vi "Trial Graphs.vi"() -> ()   [LabVIEW 2020, in "AoC 2022.lvlib"]
uses:
  <userlib>/_OpenG.lib/array/array.llb/Sort 1D Array (DBL)__ogtk.vi
  <userlib>/_OpenG.lib/array/array.llb/Index 1D Array Elements (DBL)__ogtk.vi
  AoC 2022.lvlib
  <vilib>/Analysis/NI_AAL_Geometry.lvlib
  <vilib>/4SmartMachines/Polygon Clipping/polyClipping.lvlib
panel:
  out "Polygon Set 1":T1(array[cluster])
  out "error out":errorcluster
  out "x+y 3":dbl format="%#_18f"
  out "Centroid Y":dbl format="%#_10f"
  out "Centroid X":dbl format="%#_10f"
  out "appended array":cluster{cluster{"X":dbl, "Y":dbl}[]}[](array[cluster]) {"?"."X" format="%#_17f"; "?"."Y" format="%#_17f"}
  out "x+y 2":dbl format="%#_18f"
  out "x+y":dbl format="%#_18f"
  out "element":cluster{"X":dbl, "Y":dbl} {"X" format="%#_6f"; "Y" format="%#_6f"}
  out "Array 4":T2(array[cluster])
  out "size(s) 3":i32
  out "size(s) 2":i32
  out "size(s)":i32
  in  "milliseconds to wait":u32
  out "Array 3":T2(array[cluster])
  out "Array 2":T3(array[cluster]) {"?"."Intersection X" format="%#_6f"; "?"."Intersection Y" format="%#_6f"}
  out "number of columns":i32
  out "number of rows":i32
  out "24-bit pixmap":u32[][](array[colorbox])
  out "XY Graph":cluster{"X":dbl[], "Y":dbl[]}[](graph)
  in  "Sensors":T4(c390)={{"X"=46556, "Y"=1283362}={"Beacon"={"X"=-91140, "Y"=1441882}, "Distance to Beacon"=296216.0, "Coverage Area"={"X"=[-249660.0, 46556.0, 342772.0, 46556.0, -249660.0], "Y"=[1283362.0, 987146.0, 1283362.0, 1579578.0, 1283362.0]}}, {"X"=117432, "Y"=1503889}={"Beacon"={"X"=-91140, "Y"=1441882}, "Distance to Beacon"=270579.0, "Coverage Area"={"X"=[-153147.0, 117432.0, 388011.0, 117432.0, -153147.0], "Y"=[1503889.0, 1233310.0, 1503889.0, 1774468.0, 1503889.0]}}, {"X"=117970, "Y"=37503}={"Beacon"={"X"=436611, "Y"=263737}, "Distance to Beacon"=544875.0, "Coverage Area"={"X"=[-426905.0, 117970.0, 662845.0, 117970.0, -426905.0], "Y"=[37503.0, -507372.0, 37503.0, 582378.0, 37503.0]}}, {"X"=193367, "Y"=2712458}={"Beacon"={"X"=-91140, "Y"=1441882}, "Distance to Beacon"=1555083.0, "Coverage Area"={"X"=[-1361716.0, 193367.0, 1748450.0, 193367.0, -1361716.0], "Y"=[2712458.0, 1157375.0, 2712458.0, 4267541.0, 2712458.0]}}, {"X"=220580, "Y"=684270}={"Beacon"={"X"=436611, "Y"=263737}, "Distance to Beacon"=636564.0, "Coverage Area"={"X"=[-415984.0, 220580.0, 857144.0, 220580.0, -415984.0], "Y"=[684270.0, 47706.0, 684270.0, 1320834.0, 684270.0]}}, {"X"=273443, "Y"=171076}={"Beacon"={"X"=436611, "Y"=263737}, "Distance to Beacon"=255829.0, "Coverage Area"={"X"=[17614.0, 273443.0, 529272.0, 273443.0, 17614.0], "Y"=[171076.0, -84753.0, 171076.0, 426905.0, 171076.0]}}, {"X"=480296, "Y"=3999646}={"Beacon"={"X"=1694700, "Y"=4178942}, "Distance to Beacon"=1393700.0, "Coverage Area"={"X"=[-913404.0, 480296.0, 1873996.0, 480296.0, -913404.0], "Y"=[3999646.0, 2605946.0, 3999646.0, 5393346.0, 3999646.0]}}, {"X"=608229, "Y"=955721}={"Beacon"={"X"=436611, "Y"=263737}, "Distance to Beacon"=863602.0, "Coverage Area"={"X"=[-255373.0, 608229.0, 1471831.0, 608229.0, -255373.0], "Y"=[955721.0, 92119.0, 955721.0, 1819323.0, 955721.0]}}, {"X"=766640, "Y"=26597}={"Beacon"={"X"=436611, "Y"=263737}, "Distance to Beacon"=567169.0, "Coverage Area"={"X"=[199471.0, 766640.0, 1333809.0, 766640.0, 199471.0], "Y"=[26597.0, -540572.0, 26597.0, 593766.0, 26597.0]}}, {"X"=856867, "Y"=3271314}={"Beacon"={"X"=1829362, "Y"=3182862}, "Distance to Beacon"=1060947.0, "Coverage Area"={"X"=[-204080.0, 856867.0, 1917814.0, 856867.0, -204080.0], "Y"=[3271314.0, 2210367.0, 3271314.0, 4332261.0, 3271314.0]}}, {"X"=915040, "Y"=1835970}={"Beacon"={"X"=-91140, "Y"=1441882}, "Distance to Beacon"=1400268.0, "Coverage Area"={"X"=[-485228.0, 915040.0, 2315308.0, 915040.0, -485228.0], "Y"=[1835970.0, 435702.0, 1835970.0, 3236238.0, 1835970.0]}}, {"X"=1136011, "Y"=261705}={"Beacon"={"X"=436611, "Y"=263737}, "Distance to Beacon"=701432.0, "Coverage Area"={"X"=[434579.0, 1136011.0, 1837443.0, 1136011.0, 434579.0], "Y"=[261705.0, -439727.0, 261705.0, 963137.0, 261705.0]}}, {"X"=1189379, "Y"=3999750}={"Beacon"={"X"=1694700, "Y"=4178942}, "Distance to Beacon"=684513.0, "Coverage Area"={"X"=[504866.0, 1189379.0, 1873892.0, 1189379.0, 504866.0], "Y"=[3999750.0, 3315237.0, 3999750.0, 4684263.0, 3999750.0]}}, {"X"=1531981, "Y"=3801761}={"Beacon"={"X"=1694700, "Y"=4178942}, "Distance to Beacon"=539900.0, "Coverage Area"={"X"=[992081.0, 1531981.0, 2071881.0, 1531981.0, 992081.0], "Y"=[3801761.0, 3261861.0, 3801761.0, 4341661.0, 3801761.0]}}, {"X"=1662543, "Y"=3128823}={"Beacon"={"X"=1829362, "Y"=3182862}, "Distance to Beacon"=220858.0, "Coverage Area"={"X"=[1441685.0, 1662543.0, 1883401.0, 1662543.0, 1441685.0], "Y"=[3128823.0, 2907965.0, 3128823.0, 3349681.0, 3128823.0]}}, {"X"=1728351, "Y"=2895399}={"Beacon"={"X"=1829362, "Y"=3182862}, "Distance to Beacon"=388474.0, "Coverage Area"={"X"=[1339877.0, 1728351.0, 2116825.0, 1728351.0, 1339877.0], "Y"=[2895399.0, 2506925.0, 2895399.0, 3283873.0, 2895399.0]}}, {"X"=1810202, "Y"=3423309}={"Beacon"={"X"=1829362, "Y"=3182862}, "Distance to Beacon"=259607.0, "Coverage Area"={"X"=[1550595.0, 1810202.0, 2069809.0, 1810202.0, 1550595.0], "Y"=[3423309.0, 3163702.0, 3423309.0, 3682916.0, 3423309.0]}}, {"X"=1844282, "Y"=2994285}={"Beacon"={"X"=1829362, "Y"=3182862}, "Distance to Beacon"=203497.0, "Coverage Area"={"X"=[1640785.0, 1844282.0, 2047779.0, 1844282.0, 1640785.0], "Y"=[2994285.0, 2790788.0, 2994285.0, 3197782.0, 2994285.0]}}, {"X"=1878117, "Y"=2578817}={"Beacon"={"X"=2197530, "Y"=2271330}, "Distance to Beacon"=626900.0, "Coverage Area"={"X"=[1251217.0, 1878117.0, 2505017.0, 1878117.0, 1251217.0], "Y"=[2578817.0, 1951917.0, 2578817.0, 3205717.0, 2578817.0]}}, {"X"=1894207, "Y"=1168355}={"Beacon"={"X"=2197530, "Y"=2271330}, "Distance to Beacon"=1406298.0, "Coverage Area"={"X"=[487909.0, 1894207.0, 3300505.0, 1894207.0, 487909.0], "Y"=[1168355.0, -237943.0, 1168355.0, 2574653.0, 1168355.0]}}, {"X"=2343111, "Y"=66183}={"Beacon"={"X"=2081841, "Y"=-807749}, "Distance to Beacon"=1135202.0, "Coverage Area"={"X"=[1207909.0, 2343111.0, 3478313.0, 2343111.0, 1207909.0], "Y"=[66183.0, -1069019.0, 66183.0, 1201385.0, 66183.0]}}, {"X"=2439089, "Y"=3168242}={"Beacon"={"X"=1829362, "Y"=3182862}, "Distance to Beacon"=624347.0, "Coverage Area"={"X"=[1814742.0, 2439089.0, 3063436.0, 2439089.0, 1814742.0], "Y"=[3168242.0, 2543895.0, 3168242.0, 3792589.0, 3168242.0]}}, {"X"=2482373, "Y"=2648092}={"Beacon"={"X"=2197530, "Y"=2271330}, "Distance to Beacon"=661605.0, "Coverage Area"={"X"=[1820768.0, 2482373.0, 3143978.0, 2482373.0, 1820768.0], "Y"=[2648092.0, 1986487.0, 2648092.0, 3309697.0, 2648092.0]}}, {"X"=2569893, "Y"=3911832}={"Beacon"={"X"=1694700, "Y"=4178942}, "Distance to Beacon"=1142303.0, "Coverage Area"={"X"=[1427590.0, 2569893.0, 3712196.0, 2569893.0, 1427590.0], "Y"=[3911832.0, 2769529.0, 3911832.0, 5054135.0, 3911832.0]}}, {"X"=2605308, "Y"=2023938}={"Beacon"={"X"=2197530, "Y"=2271330}, "Distance to Beacon"=655170.0, "Coverage Area"={"X"=[1950138.0, 2605308.0, 3260478.0, 2605308.0, 1950138.0], "Y"=[2023938.0, 1368768.0, 2023938.0, 2679108.0, 2023938.0]}}, {"X"=3047883, "Y"=3301452}={"Beacon"={"X"=3537901, "Y"=3368697}, "Distance to Beacon"=557263.0, "Coverage Area"={"X"=[2490620.0, 3047883.0, 3605146.0, 3047883.0, 2490620.0], "Y"=[3301452.0, 2744189.0, 3301452.0, 3858715.0, 3301452.0]}}, {"X"=3056788, "Y"=2626224}={"Beacon"={"X"=3355914, "Y"=2862466}, "Distance to Beacon"=535368.0, "Coverage Area"={"X"=[2521420.0, 3056788.0, 3592156.0, 3056788.0, 2521420.0], "Y"=[2626224.0, 2090856.0, 2626224.0, 3161592.0, 2626224.0]}}, {"X"=3199067, "Y"=2194575}={"Beacon"={"X"=3748004, "Y"=2000000}, "Distance to Beacon"=743512.0, "Coverage Area"={"X"=[2455555.0, 3199067.0, 3942579.0, 3199067.0, 2455555.0], "Y"=[2194575.0, 1451063.0, 2194575.0, 2938087.0, 2194575.0]}}, {"X"=3329538, "Y"=3016377}={"Beacon"={"X"=3355914, "Y"=2862466}, "Distance to Beacon"=180287.0, "Coverage Area"={"X"=[3149251.0, 3329538.0, 3509825.0, 3329538.0, 3149251.0], "Y"=[3016377.0, 2836090.0, 3016377.0, 3196664.0, 3016377.0]}}, {"X"=3399994, "Y"=700264}={"Beacon"={"X"=3748004, "Y"=2000000}, "Distance to Beacon"=1647746.0, "Coverage Area"={"X"=[1752248.0, 3399994.0, 5047740.0, 3399994.0, 1752248.0], "Y"=[700264.0, -947482.0, 700264.0, 2348010.0, 700264.0]}}, {"X"=3598024, "Y"=3322247}={"Beacon"={"X"=3537901, "Y"=3368697}, "Distance to Beacon"=106573.0, "Coverage Area"={"X"=[3491451.0, 3598024.0, 3704597.0, 3598024.0, 3491451.0], "Y"=[3322247.0, 3215674.0, 3322247.0, 3428820.0, 3322247.0]}}, {"X"=3604375, "Y"=3668021}={"Beacon"={"X"=3537901, "Y"=3368697}, "Distance to Beacon"=365798.0, "Coverage Area"={"X"=[3238577.0, 3604375.0, 3970173.0, 3604375.0, 3238577.0], "Y"=[3668021.0, 3302223.0, 3668021.0, 4033819.0, 3668021.0]}}, {"X"=3620241, "Y"=2904998}={"Beacon"={"X"=3355914, "Y"=2862466}, "Distance to Beacon"=306859.0, "Coverage Area"={"X"=[3313382.0, 3620241.0, 3927100.0, 3620241.0, 3313382.0], "Y"=[2904998.0, 2598139.0, 2904998.0, 3211857.0, 2904998.0]}}, {"X"=3680413, "Y"=2477027}={"Beacon"={"X"=3748004, "Y"=2000000}, "Distance to Beacon"=544618.0, "Coverage Area"={"X"=[3135795.0, 3680413.0, 4225031.0, 3680413.0, 3135795.0], "Y"=[2477027.0, 1932409.0, 2477027.0, 3021645.0, 2477027.0]}}, {"X"=3741660, "Y"=3959257}={"Beacon"={"X"=3537901, "Y"=3368697}, "Distance to Beacon"=794319.0, "Coverage Area"={"X"=[2947341.0, 3741660.0, 4535979.0, 3741660.0, 2947341.0], "Y"=[3959257.0, 3164938.0, 3959257.0, 4753576.0, 3959257.0]}}, {"X"=3891093, "Y"=2110588}={"Beacon"={"X"=3748004, "Y"=2000000}, "Distance to Beacon"=253677.0, "Coverage Area"={"X"=[3637416.0, 3891093.0, 4144770.0, 3891093.0, 3637416.0], "Y"=[2110588.0, 1856911.0, 2110588.0, 2364265.0, 2110588.0]}}, {"X"=3951385, "Y"=3125577}={"Beacon"={"X"=3537901, "Y"=3368697}, "Distance to Beacon"=656604.0, "Coverage Area"={"X"=[3294781.0, 3951385.0, 4607989.0, 3951385.0, 3294781.0], "Y"=[3125577.0, 2468973.0, 3125577.0, 3782181.0, 3125577.0]}}, {"X"=3992558, "Y"=1933059}={"Beacon"={"X"=3748004, "Y"=2000000}, "Distance to Beacon"=311495.0, "Coverage Area"={"X"=[3681063.0, 3992558.0, 4304053.0, 3992558.0, 3681063.0], "Y"=[1933059.0, 1621564.0, 1933059.0, 2244554.0, 1933059.0]}}}
  out "Array":T5(array[cluster])
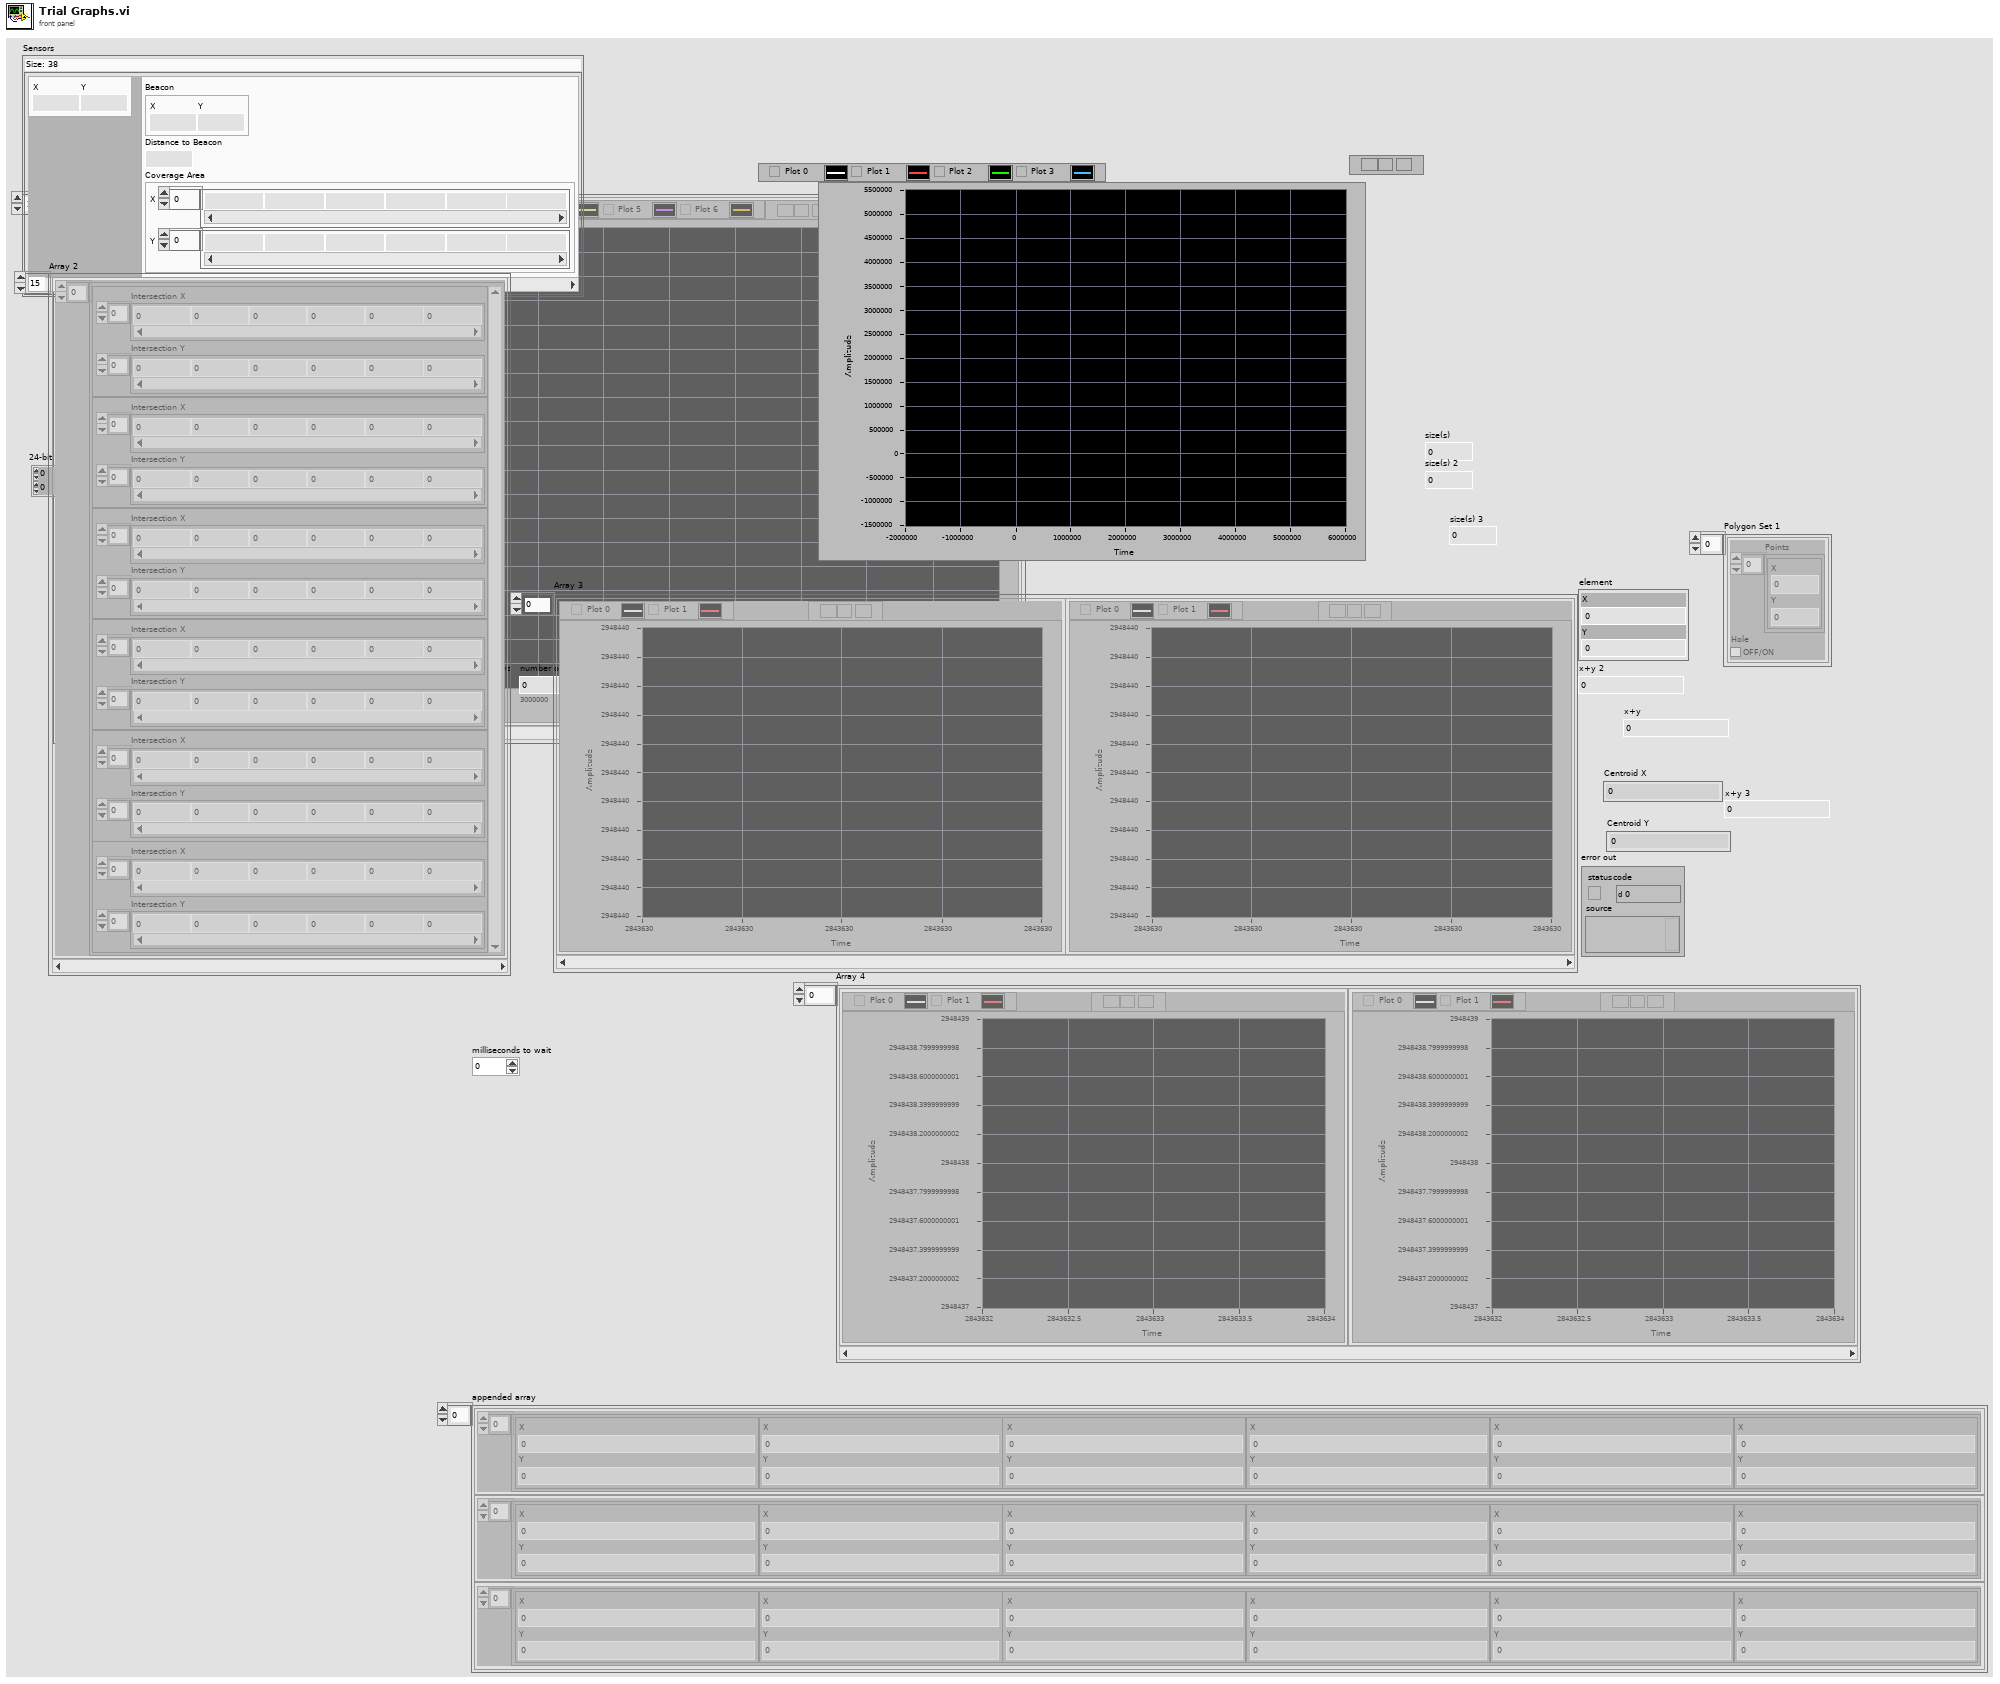
[diagram p1: front panel]
types:
  T1 = cluster{"Points":cluster{"X":dbl, "Y":dbl}[], "Hole":bool}[]
  T2 = cluster{"XY Graph 2":cluster{"X":dbl, "Y":dbl}[]}[]
  T3 = cluster{cluster{"Intersection X":dbl[], "Intersection Y":dbl[]}[]}[]
  T4 = map{cluster{"X":i32, "Y":i32}, cluster{"Beacon":cluster{"X":i32, "Y":i32}, "Distance to Beacon":dbl, "Coverage Area":cluster{"X":dbl[], "Y":dbl[]}}}
  T5 = cluster{"XY Graph 2":cluster{"Intersection X":dbl[], "Intersection Y":dbl[]}[]}[]
  T6 = enum16{"Intersection", "Union", "Difference", "Xor"}
  T7 = cluster{"left":i16, "top":i16, "right":i16, "bottom":i16}
  T8 = cluster{"Intersection X":dbl[], "Intersection Y":dbl[]}
  T9 = cluster{"Sorted Array out":dbl[], "elements":dbl[]}
  T10 = cluster{"Sorted Array out":dbl[], "elements":dbl[]}[]
  T11 = cluster{cluster{"Sorted Array out":dbl[], "elements":dbl[]}[]}
  T12 = cluster{"Points":cluster{"X":dbl, "Y":dbl}[], "Hole":bool}
  T13 = typedef "imagedata.ctl" = cluster{"image type":i32, "image depth":i32, "image":u8[], "mask":u8[], "colors":u32[], "Rectangle":cluster{"left":i16, "top":i16, "right":i16, "bottom":i16}}
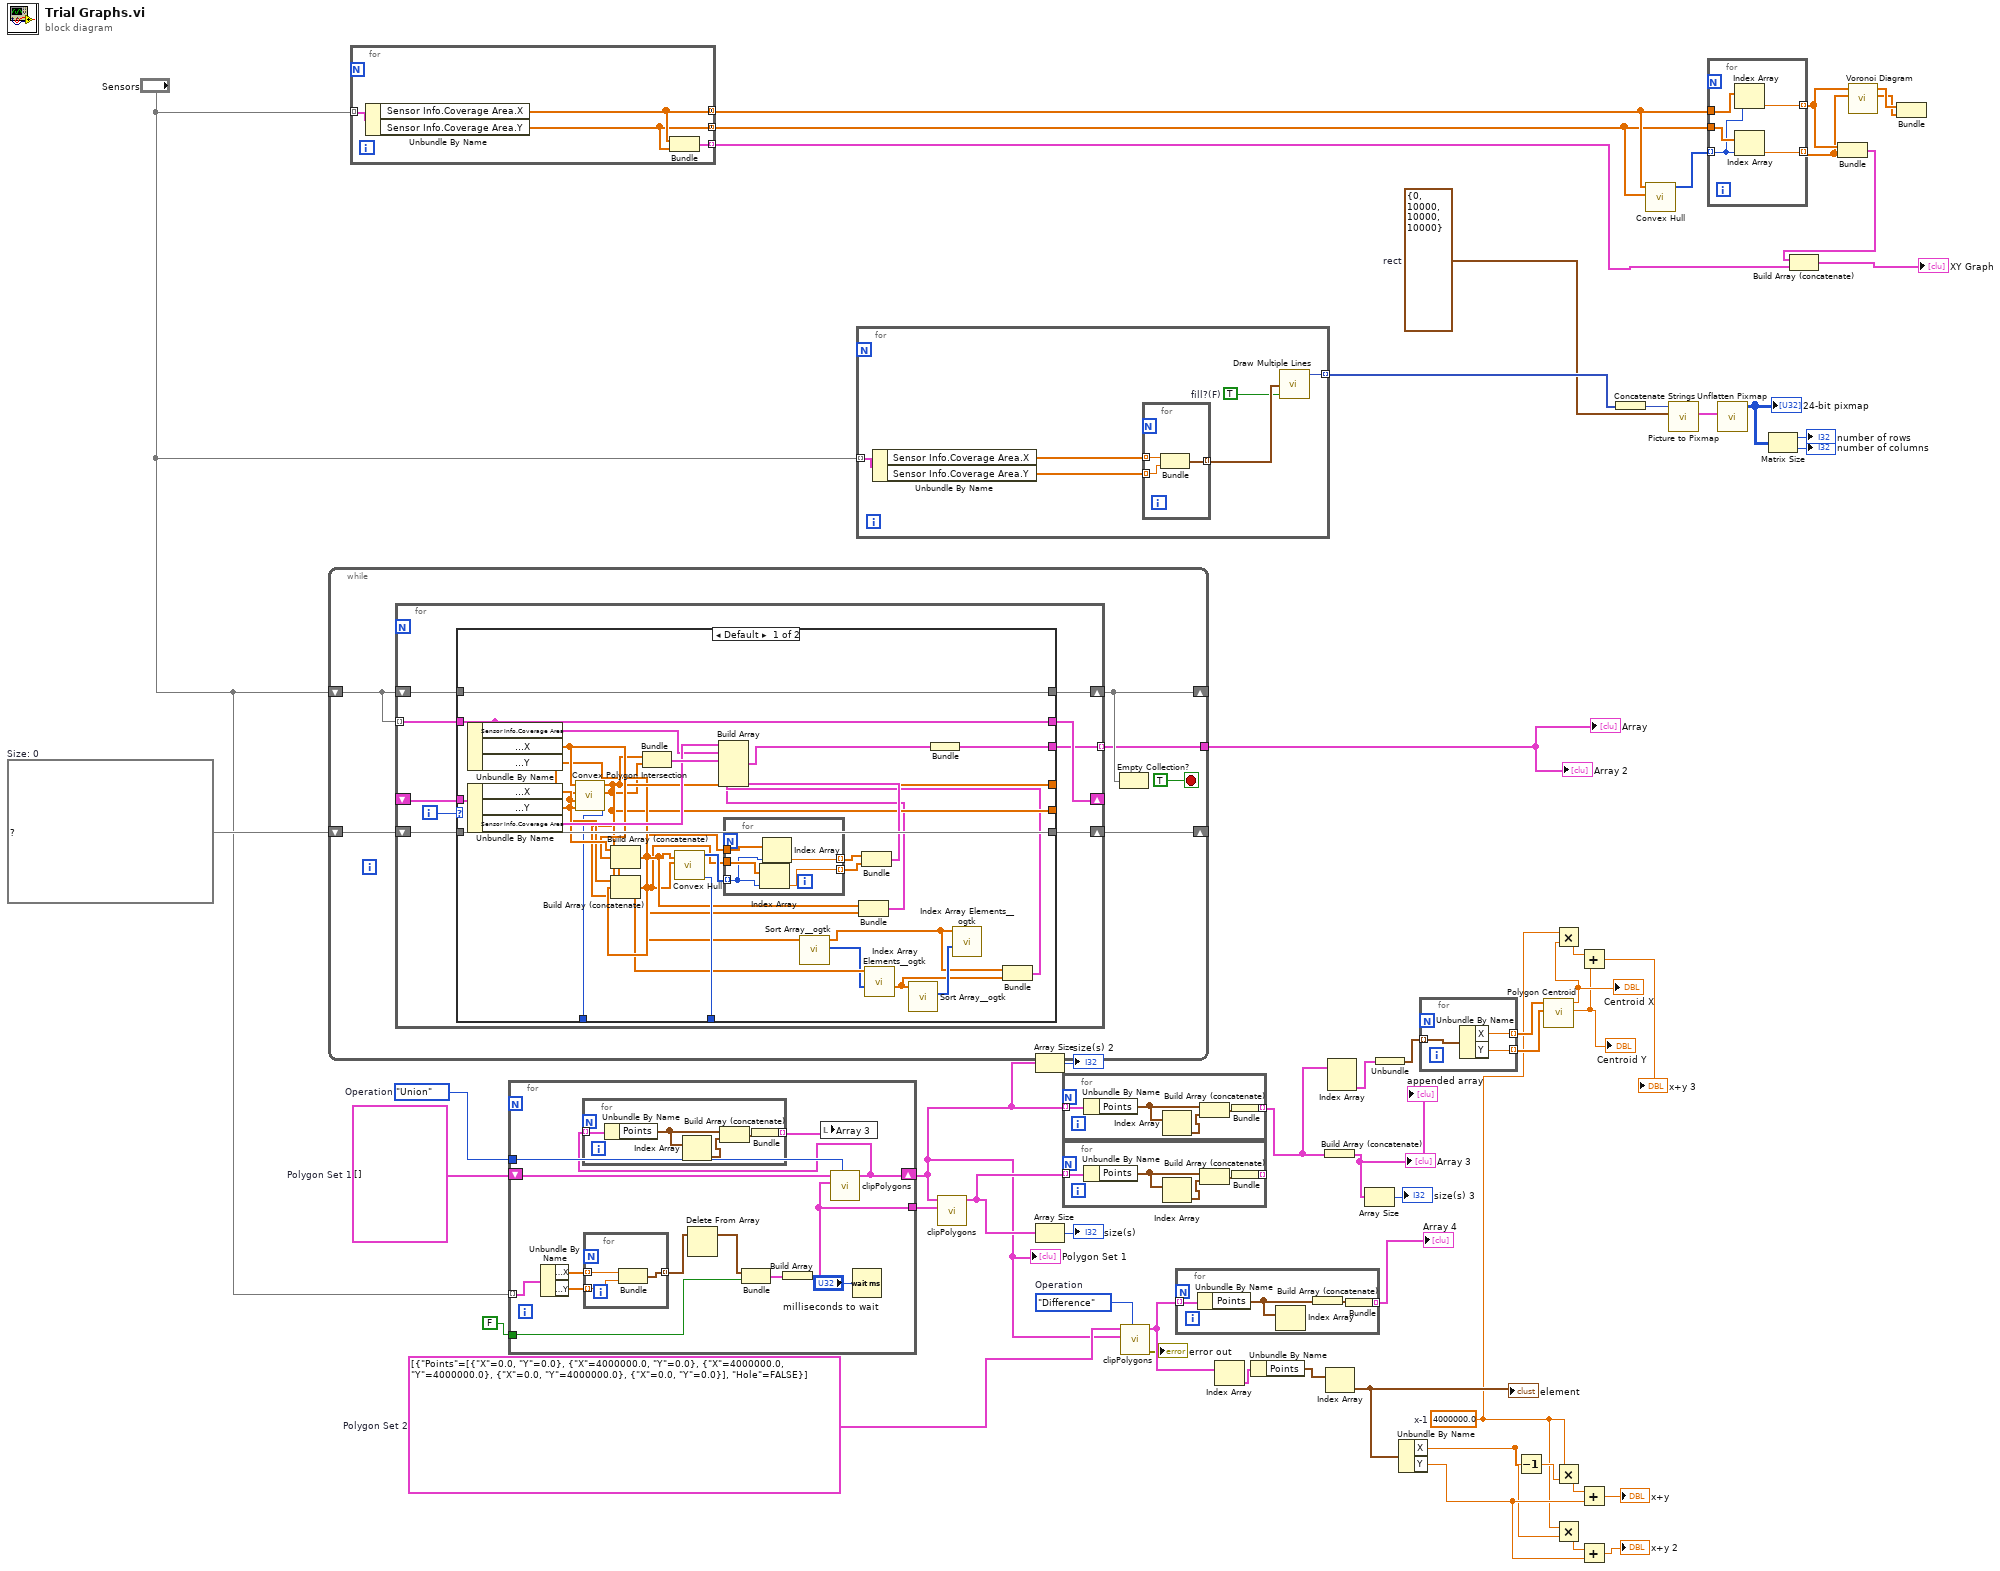
[diagram p0: block diagram]
diagram:
  w4 = 4000000.0  # x-1
  w31 = T1 [{"Points"=[{"X"=0.0, "Y"=0.0}, {"X"=4000000.0, "Y"=0.0}, {"X"=4000000.0, "Y"=4000000.0}, {"X"=0.0, "Y"=4000000.0}, {"X"=0.0, "Y"=0.0}], "Hole"=FALSE}]  # Polygon Set 2
  w32 = T6."Difference"  # Operation
  w35 = T6."Union"  # Operation
  w36 = T1 []  # Polygon Set 1
  w38 = map{i32, cluster{"X":dbl[], "Y":dbl[]}} {}  # Size: 0
  w39 = T7 {"left"=0, "top"=10000, "right"=10000, "bottom"=10000}  # rect
  n1 = while {
    shift-right: [w60] -> _
    shift-left: "Sensors" -> [w61]
    shift-right: [w58] -> _
    shift-left: w38 -> [w59]
    tunnel: [w56] -> w37
    stop <- TRUE stop-if-true
    n2 = for {
      shift-right: [w68] -> w60
      shift-left: w61 -> [w70]
      tunnel: w61 -> [w66] mode=indexing
      shift-right: [w63] -> w58
      shift-left: w59 -> [w64]
      shift-right: [w67] -> _
      shift-left: _ -> [w65]
      tunnel: [w62] -> w56 mode=indexing
      i -> [w69]
      n3 = case shown="Default" w69 {
        tunnel: w70 -> [w99 w107]
        tunnel: [w99 w107] -> w68
        tunnel: [w97 w106] -> w67
        tunnel: w66 -> [w97 w106]
        tunnel: w65 -> [w98 _]
        tunnel: w64 -> [w96 w105]
        tunnel: [w96 w105] -> w63
        tunnel: [w86 _] -> _
        tunnel: [w83 _] -> _
        tunnel: [w82 _] -> _
        tunnel: [w81 _] -> _
        tunnel: [w79 _] -> w62
        frame Default {
          n4 = Unbundle By Name(w97) -> ("Sensor Info.Coverage Area"=w93:cluster{"X":dbl[], "Y":dbl[]}, "Sensor Info.Coverage Area.X"=w87:dbl[], "Sensor Info.Coverage Area.Y"=w84:dbl[])
          n5 = Unbundle By Name(w98) -> ("Sensor Info.Coverage Area.X"=w88:dbl[], "Sensor Info.Coverage Area.Y"=w85:dbl[], "Sensor Info.Coverage Area"=w94:cluster{"X":dbl[], "Y":dbl[]})
          n6 = call <vilib>:"Convex Polygon Intersection.vi"("Y 2"=w85, "X 2"=w88, "Y 1"=w84, "X 1"=w87) -> ("error"=w81:i32, "Intersection Y"=w83:dbl[], "Intersection X"=w86:dbl[])  [unwired: 5 in]
          n7 = Build Array (concatenate)(w88, w87, w86) -> (w78:dbl[])
          n8 = Build Array (concatenate)(w85, w84, w83) -> (w77:dbl[])
          n9 = Bundle("Intersection X"=w86, "Intersection Y"=w83) -> (w95:T8)  [unwired: 1 in]
          n10 = call <vilib>:"Convex Hull.vi"("Y"=w77, "X"=w78) -> ("error"=w82:i32, "Convex Hull"=w92:i32[])  [unwired: 8 in]
          n11 = for {
            tunnel: w92 -> [w102] mode=indexing
            tunnel: w78 -> [w104]
            tunnel: w77 -> [w103]
            tunnel: [w101] -> w91 mode=indexing
            tunnel: [w100] -> w90 mode=indexing
            n12 = Index Array(array=w103, index=w102) -> (element=w100:dbl)
            n13 = Index Array(array=w104, index=w102) -> (element=w101:dbl)
          }
          n14 = call-poly <userlib>:"Sort Array__ogtk.vi"("Array in"=w78) -> ("Sorted Pointers"=w76:i32[], "Sorted Array out"=w72:dbl[])  [unwired: 9 in]
          n15 = Bundle(w78, w77) -> (w71:cluster{dbl[], dbl[]})  [unwired: 1 in]
          n16 = Bundle(w91, w90) -> (w89:cluster{dbl[], dbl[]})  [unwired: 1 in]
          n17 = call-poly <userlib>:"Index Array Elements__ogtk.vi"("indices"=w76, "array"=w77) -> ("elements"=w73:dbl[])  [unwired: 9 in]
          n18 = call-poly <userlib>:"Sort Array__ogtk.vi"("Array in"=w73) -> ("Sorted Pointers"=w75:i32[])  [unwired: 9 in, 1 out]
          n19 = call-poly <userlib>:"Index Array Elements__ogtk.vi"("indices"=w75, "array"=w72) -> ()  [unwired: 9 in, 1 out]
          n20 = Bundle("Sorted Array out"=w72, "elements"=w73) -> (w74:T9)  [unwired: 1 in]
          n21 = Build Array(w94, w93, w95, w89, w74, w71) -> (w80:T10)
          n22 = Bundle(w80) -> (w79:T11)  [unwired: 1 in]
        }
        frame 0 {
        }
      }
    }
    n23 = Empty Collection?(1:w60) -> ()  [unwired: 1 out]
  }
  "Array" <- w37
  "Array 2" <- w37
  n24 = for {
    tunnel: "Sensors" -> [w111] mode=indexing
    tunnel: [w109] -> w54 mode=concatenating
    tunnel: [w108] -> w53 mode=concatenating
    tunnel: [w110] -> w50 mode=indexing
    n25 = Unbundle By Name(w111) -> ("Sensor Info.Coverage Area.X"=w109:dbl[], "Sensor Info.Coverage Area.Y"=w108:dbl[])
    n26 = Bundle("X"=w109, "Y"=w108) -> (w110:cluster{"X":dbl[], "Y":dbl[]})  [unwired: 1 in]
  }
  n27 = for {
    shift-right: [w117] -> w24
    shift-left: w36 -> [w124]
    tunnel: w35 -> [w123]
    tunnel: "Sensors" -> [w122] mode=indexing
    tunnel: FALSE -> [w119]
    tunnel: [w114] -> w30
    n28 = Unbundle By Name(w122) -> ("Sensor Info.Coverage Area.X"=w121:dbl[], "Sensor Info.Coverage Area.Y"=w120:dbl[])
    n29 = for {
      tunnel: w121 -> [w132] mode=indexing
      tunnel: w120 -> [w131] mode=indexing
      tunnel: [w130] -> w113 mode=indexing
      n30 = Bundle("X"=w132, "Y"=w131) -> (w130:cluster{"X":dbl, "Y":dbl})  [unwired: 1 in]
    }
    n31 = Delete From Array(array=w113) -> (array with subset deleted=w112:cluster{"X":dbl, "Y":dbl}[])  [unwired: 2 in, 1 out]
    n32 = Bundle(w112, w119) -> (w118:cluster{cluster{"X":dbl, "Y":dbl}[], bool})  [unwired: 1 in]
    n33 = Build Array(w118) -> (w114:cluster{cluster{"X":dbl, "Y":dbl}[], bool}[])
    n34 = call <vilib>:"clipPolygons.vi"("Operation"=w123, "Polygon Set 2"=w114, "Polygon Set 1"=w124) -> ("Polygon Set Out"=w117:T1)  [unwired: 7 in, 1 out]
    n35 = for {
      tunnel: w117 -> [w129] mode=indexing
      tunnel: [w128] -> w116 mode=indexing
      n36 = Unbundle By Name(w129) -> ("Points"=w127:cluster{"X":dbl, "Y":dbl}[])
      n37 = Index Array(array=w127) -> (element=w125:cluster{"X":dbl, "Y":dbl})  [unwired: 1 in]
      n38 = Build Array (concatenate)(w127, w125) -> (w126:cluster{"X":dbl, "Y":dbl}[])
      n39 = Bundle(w126) -> (w128:cluster{cluster{"X":dbl, "Y":dbl}[]})  [unwired: 1 in]
    }
    n40 = local write "Array 3"(w116) -> ()
    n41 = Wait (ms)(milliseconds to wait="milliseconds to wait") -> ()  [unwired: 1 out]
  }
  "Polygon Set 1" <- w24
  n42 = for {
    tunnel: "Sensors" -> [w138] mode=indexing
    tunnel: [w134] -> w45 mode=indexing
    w133 = TRUE  # fill?(F)
    n43 = Unbundle By Name(w138) -> ("Sensor Info.Coverage Area.X"=w137:dbl[], "Sensor Info.Coverage Area.Y"=w136:dbl[])
    n44 = for {
      tunnel: w137 -> [w141] mode=indexing
      tunnel: w136 -> [w140] mode=indexing
      tunnel: [w139] -> w135 mode=indexing
      n45 = Bundle("X"=w141, "Y"=w140) -> (w139:cluster{"X":dbl, "Y":dbl})  [unwired: 1 in]
    }
    n46 = call <vilib>:"Draw Multiple Lines.vi"("line endpoints"=w135, "fill?(F)"=w133) -> ("new picture"=w134:picture)  [unwired: 7 in]
  }
  n47 = call <vilib>:"clipPolygons.vi"("Polygon Set 2"=w30, "Polygon Set 1"=w24) -> ("Polygon Set Out"=w29:T1)  [unwired: 8 in, 1 out]
  n48 = Array Size(array=w24) -> (size(s)=→"size(s) 2":i32)
  n49 = Array Size(array=w29) -> (size(s)=→"size(s)":i32)
  n50 = for {
    tunnel: w24 -> [w146] mode=indexing
    tunnel: [w145] -> w11 mode=indexing
    n51 = Unbundle By Name(w146) -> ("Points"=w144:cluster{"X":dbl, "Y":dbl}[])
    n52 = Index Array(array=w144) -> (element=w142:cluster{"X":dbl, "Y":dbl})  [unwired: 1 in]
    n53 = Build Array (concatenate)(w144, w142) -> (w143:cluster{"X":dbl, "Y":dbl}[])
    n54 = Bundle(w143) -> (w145:cluster{cluster{"X":dbl, "Y":dbl}[]})  [unwired: 1 in]
  }
  n55 = for {
    tunnel: w29 -> [w151] mode=indexing
    tunnel: [w150] -> _ mode=indexing
    n56 = Unbundle By Name(w151) -> ("Points"=w149:cluster{"X":dbl, "Y":dbl}[])
    n57 = Index Array(array=w149) -> (element=w147:cluster{"X":dbl, "Y":dbl})  [unwired: 1 in]
    n58 = Build Array (concatenate)(w149, w147) -> (w148:cluster{"X":dbl, "Y":dbl}[])
    n59 = Bundle(w148) -> (w150:cluster{cluster{"X":dbl, "Y":dbl}[]})  [unwired: 1 in]
  }
  n60 = call <vilib>:"clipPolygons.vi"("Operation"=w32, "Polygon Set 2"=w24, "Polygon Set 1"=w31) -> ("error out"=→"error out":errorcluster, "Polygon Set Out"=w22:T1)  [unwired: 7 in]
  n61 = for {
    tunnel: w22 -> [w155] mode=indexing
    tunnel: [w154] -> w23 mode=indexing
    n62 = Unbundle By Name(w155) -> ("Points"=w153:cluster{"X":dbl, "Y":dbl}[])
    n63 = Index Array(array=w153) -> ()  [unwired: 1 in, 1 out]
    n64 = Build Array (concatenate)(w153) -> (w152:cluster{"X":dbl, "Y":dbl}[])
    n65 = Bundle(w152) -> (w154:cluster{cluster{"X":dbl, "Y":dbl}[]})  [unwired: 1 in]
  }
  "Array 4" <- w23
  n66 = Index Array(array=w22) -> (element=w21:T12)  [unwired: 1 in]
  n67 = Unbundle By Name(w21) -> ("Points"=w20:cluster{"X":dbl, "Y":dbl}[])
  n68 = Build Array (concatenate)(w11) -> (w25:cluster{cluster{"X":dbl, "Y":dbl}[]}[])
  "Array 3" <- w25
  "appended array" <- w25
  n69 = Index Array(array=w20) -> (element=w19:cluster{"X":dbl, "Y":dbl})  [unwired: 1 in]
  "element" <- w19
  n70 = Index Array(array=w11) -> (element #2=w10:cluster{cluster{"X":dbl, "Y":dbl}[]})  [unwired: 2 in, 1 out]
  n71 = Array Size(array=w25) -> (size(s)=→"size(s) 3":i32)
  n72 = Unbundle(w10) -> (w9:cluster{"X":dbl, "Y":dbl}[])
  n73 = Unbundle By Name(w19) -> ("X"=w13:dbl, "Y"=w14:dbl)
  n74 = for {
    tunnel: w9 -> [w158] mode=indexing
    tunnel: [w157] -> w8 mode=indexing
    tunnel: [w156] -> w7 mode=indexing
    n75 = Unbundle By Name(w158) -> ("X"=w157:dbl, "Y"=w156:dbl)
  }
  n76 = Decrement(x=w13) -> (x-1=w18:dbl)
  n77 = call <vilib>:"Polygon Centroid.vi"("Y"=w7, "X"=w8) -> ("Centroid Y"=w3:dbl, "Centroid X"=w5:dbl)  [unwired: 7 in, 1 out]
  "Centroid X" <- w5
  "Centroid Y" <- w3
  n78 = Multiply(x=w4, y=w5) -> (x*y=w6:dbl)
  n79 = Multiply(x=w4, y=w18) -> (x*y=w17:dbl)
  n80 = Multiply(x=w4, y=w13) -> (x*y=w15:dbl)
  n81 = Add(x=w6, y=w3) -> (x+y=→"x+y 3":dbl)
  n82 = Add(x=w17, y=w14) -> (x+y=→"x+y":dbl)
  n83 = Add(x=w15, y=w14) -> (x+y=→"x+y 2":dbl)
  n84 = Concatenate Strings(w45) -> (w44:picture)
  n85 = call <vilib>:"Convex Hull.vi"("Y"=w53, "X"=w54) -> ("Convex Hull"=w55:i32[])  [unwired: 8 in, 1 out]
  n86 = call <vilib>:"Picture to Pixmap.vi"("rect"=w39, "picture"=w44) -> ("image data"=w43:T13)  [unwired: 8 in, 1 out]
  n87 = for {
    tunnel: w54 -> [w163]
    tunnel: w53 -> [w162]
    tunnel: w55 -> [w161] mode=indexing
    tunnel: [w160] -> w49 mode=indexing
    tunnel: [w159] -> w48 mode=indexing
    n88 = Index Array(array=w163, index=w161) -> (element=w160:dbl)
    n89 = Index Array(array=w162, index=w161) -> (element=w159:dbl)
  }
  n90 = call <vilib>:"Unflatten Pixmap.vi"("image data"=w43) -> ("24-bit pixmap"=w42:u32[][])  [unwired: 4 in, 6 out]
  "24-bit pixmap" <- w42
  n91 = Matrix Size(0:w42) -> (1:→"number of rows":i32, 2:→"number of columns":i32)
  n92 = Bundle(w49, w48) -> (w51:cluster{dbl[], dbl[]})  [unwired: 1 in]
  n93 = Build Array (concatenate)(w51, w50) -> (→"XY Graph":cluster{"X":dbl[], "Y":dbl[]}[])
  n94 = call <vilib>:"Voronoi Diagram.vi"("Y"=w48, "X"=w49) -> ("Voronoi Y"=w46:dbl[], "Voronoi X"=w47:dbl[])  [unwired: 6 in, 2 out]
  n95 = Bundle("Voronoi X"=w47, "Voronoi Y"=w46) -> ()  [unwired: 1 in, 1 out]
